vi "Camera Positioning 2.vi"(8 "Aim":bool, 10 "Y Position":dbl=1.0 min=1.0 max=20.0 step=0.1, 11 "X Position":dbl min=-1.0 max=1.0 step=0.01) -> (0 "Aim Finished":bool, 2 "Fwd/Rev Out":dbl, 3 "Left/Right Out":dbl)   [LabVIEW 2015]
panel:
  out "Numeric 2":dbl
  out "Numeric":dbl
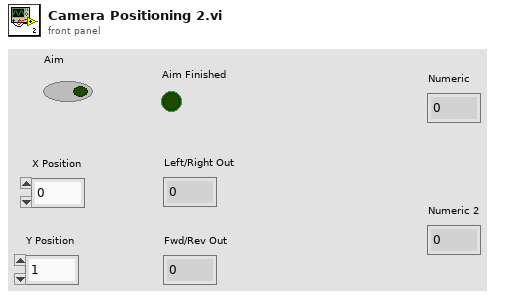
[diagram p1: front panel]
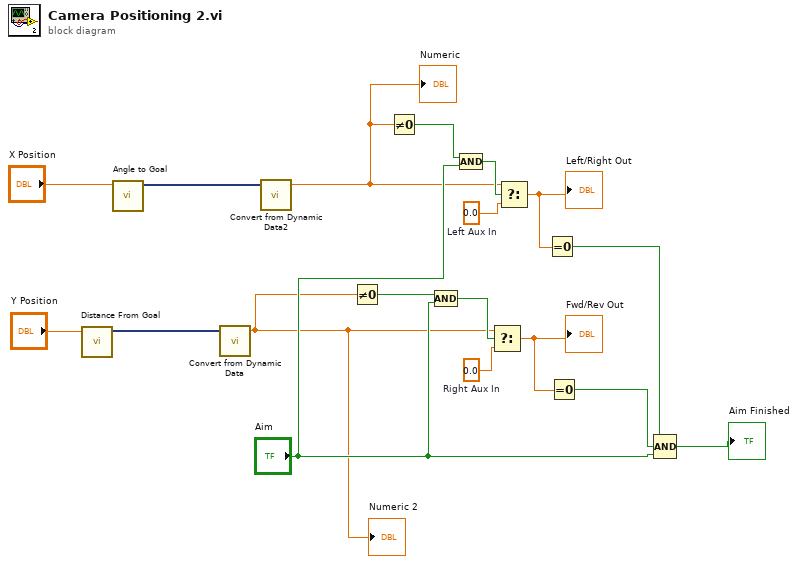
[diagram p0: block diagram]
diagram:
  w18 = 0.0  # Left Aux In
  w17 = 0.0  # Right Aux In
  n1 = call "Distance From Goal"("Signals"="Y Position") -> ("Scaled Signals"=w10:dynamicdata)  [unwired: 9 in, 1 out]
  n2 = call "Angle to Goal"("Signals"="X Position") -> ("Scaled Signals"=w9:dynamicdata)  [unwired: 9 in, 1 out]
  n3 = call "Convert from Dynamic Data"("Dynamic Data Type"=w10) -> ("Scalar"=w1:dbl)  [unwired: 3 in]
  "Numeric 2" <- w1
  n4 = call "Convert from Dynamic Data2"("Dynamic Data Type"=w9) -> ("Scalar"=w2:dbl)  [unwired: 3 in]
  "Numeric" <- w2
  n5 = Not Equal To 0?(x=w1) -> (x != 0?=w15:bool)
  n6 = Not Equal To 0?(x=w2) -> (x != 0?=w14:bool)
  n7 = Compound Arithmetic op=AND(w15, "Aim") -> (w16:bool)
  n8 = Compound Arithmetic op=AND(w14, "Aim") -> (w13:bool)
  n9 = Select(t=w1, s=w16, f=w17) -> (s? t:f=w3:dbl)
  "Fwd/Rev Out" <- w3
  n10 = Select(t=w2, s=w13, f=w18) -> (s? t:f=w4:dbl)
  "Left/Right Out" <- w4
  n11 = Equal To 0?(x=w4) -> (x = 0?=w5:bool)
  n12 = Equal To 0?(x=w3) -> (x = 0?=w6:bool)
  n13 = Compound Arithmetic op=AND(w5, w6, "Aim") -> (→"Aim Finished":bool)
